vi "Stop.vi"(6 "Teller":refnum<class "Teller.lvclass">, 9 "Parent Stopped":bool, 10 "Safe Stop":bool=TRUE, 11 "Stop in":refnum<class "Stop.lvclass">) -> (0 "Error out":errorcluster, 3 "Stop out":refnum<class "Stop.lvclass">)   [LabVIEW 2025, in "jettl.lvlib" / "Stop Msg.lvlib" / "Stop.lvclass"]
uses:
  Stop.lvclass
  Teller/Teller/Teller.lvclass
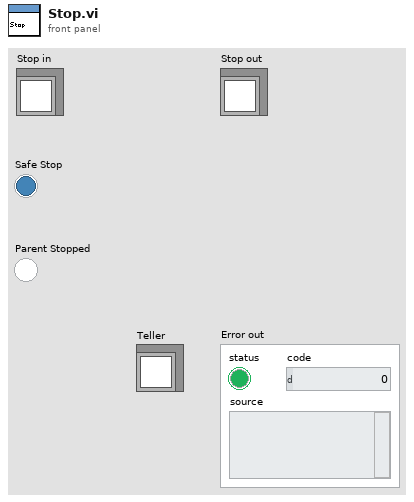
[diagram p1: front panel]
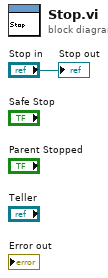
[diagram p0: block diagram]
diagram:
  "Stop out" <- "Stop in"
